vi "PantherLAB_Log - Duplicate DQMH Event.vi"(6 "Round Trip Broadcast Name":string, 7 "Destination Module":T1, 9 "New Event Name":string, 10 "Event Info (Existing)":T3={"Event VI Path"=path "", "Argument Path"=path "", "Wait Argument Path"=path "", "Event Arg Owner"=-1, "Event Name"="", "Type"=enum."Request"}, 11 "Source Module":T1) -> (0 "error out":errorcluster)   [LabVIEW 2016]
doc: "_____\nCreated using DQMH Framework: Event Scripter 7.1.0.1450."
uses:
  <vilib>/Delacor/Delacor QMH/Libraries/_Scripting Support/Module Info--cluster.ctl
  <vilib>/Delacor/Delacor QMH/Libraries/_Scripting Support/Module Type--enum.ctl
  <vilib>/Delacor/Delacor QMH/Libraries/_Scripting Support/Event Info (Existing)--cluster.ctl
  Program Files (x86)/National Instruments/LabVIEW 2016/project/Delacor/DQMH/_DQMH Remove Event/Event Type (All Permutations)--enum.ctl
  PantherLAB Scripting Hooks/PantherLAB_Scripting.lvlib
  <vilib>/Delacor/Delacor QMH/Libraries/_Scripting Support/dqmh_lib_DQMH Scripting Support.lvlib
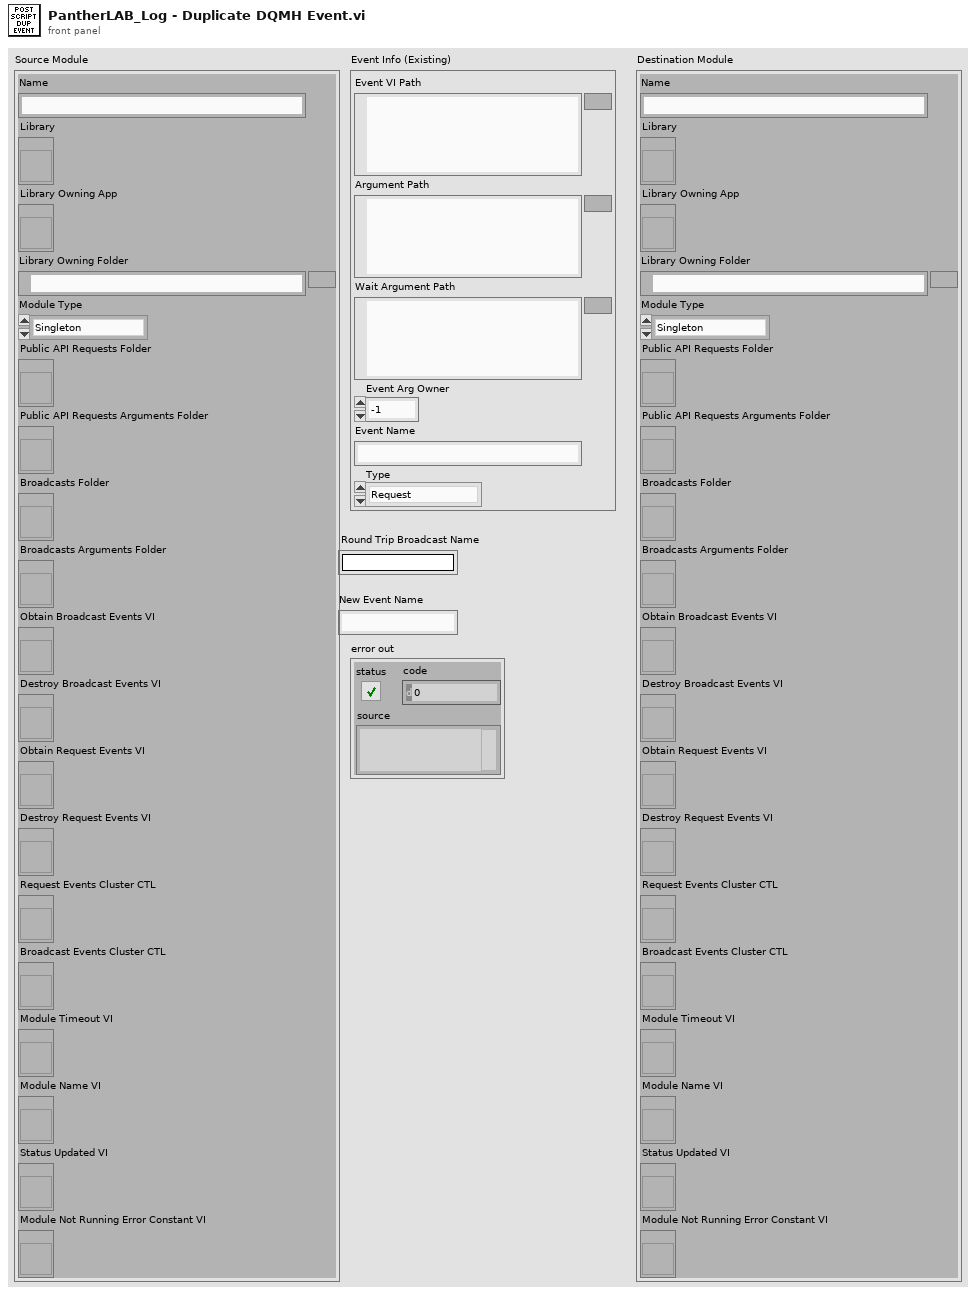
[diagram p1: front panel]
types:
  T1 = typedef "dqmh_lib_DQMH Scripting Support.lvlib/Module Info--cluster.ctl" = cluster{"Name":string, "Library":refnum<vi>, "Library Owning App":refnum<vi>, "Library Owning Folder":path, "Module Type":T2, "Public API Requests Folder":refnum<vi>, "Public API Requests Arguments Folder":refnum<vi>, "Broadcasts Folder":refnum<vi>, "Broadcasts Arguments Folder":refnum<vi>, "Obtain Broadcast Events VI":refnum<vi>, "Destroy Broadcast Events VI":refnum<vi>, "Obtain Request Events VI":refnum<vi>, "Destroy Request Events VI":refnum<vi>, "Request Events Cluster CTL":refnum<vi>, "Broadcast Events Cluster CTL":refnum<vi>, "Module Timeout VI":refnum<vi>, "Module Name VI":refnum<vi>, "Status Updated VI":refnum<vi>, "Module Not Running Error Constant VI":refnum<vi>}
  T2 = typedef "dqmh_lib_DQMH Scripting Support.lvlib/Module Type--enum.ctl" = enum16{"Singleton", "Cloneable"}
  T3 = typedef "dqmh_lib_DQMH Scripting Support.lvlib/Event Info (Existing)--cluster.ctl" = cluster{"Event VI Path":path, "Argument Path":path, "Wait Argument Path":path, "Event Arg Owner":i32, "Event Name":string, "Type":T4}
  T4 = typedef "dqmh_lib_DQMH Scripting Support.lvlib/Event Type (All Permutations)--enum.ctl" = enum16{"Request", "Broadcast", "Both", "Request (no Wait)", "Request and Wait", "Request (Private)", "Request (Local Instance)"}
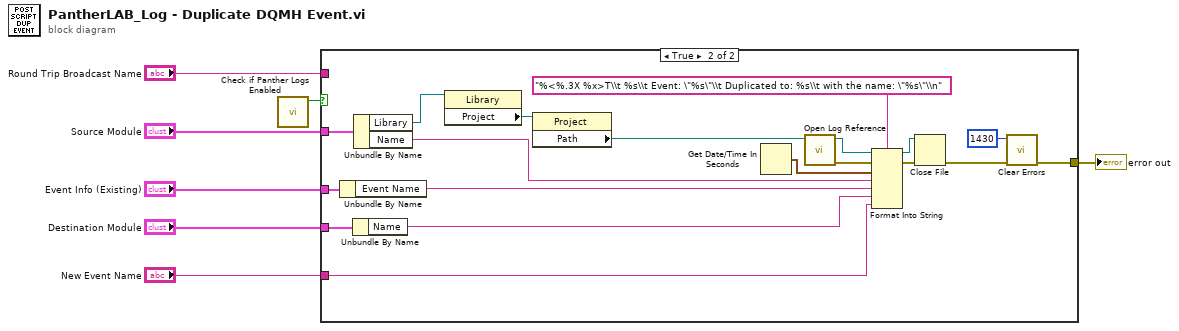
[diagram p0: block diagram]
diagram:
  n1 = call "Check if Panther Logs Enabled.vi"() -> ("PantherLogs Enabled?"=w6:bool)  [unwired: 11 in]
  n2 = case shown="True" w6 {
    tunnel: [_ w9] -> w7
    tunnel: "Source Module" -> [_ w23]
    tunnel: "Destination Module" -> [_ w13]
    tunnel: "Event Info (Existing)" -> [_ w15]
    tunnel: "New Event Name" -> [_ w11]
    tunnel: "Round Trip Broadcast Name" -> [_ _]
    frame False {
    }
    frame True {
      n3 = Unbundle By Name(w15) -> ("Event Name"=w14:string)
      n4 = Unbundle By Name(w13) -> ("Name"=w12:string)
      n5 = Unbundle By Name(w23) -> ("Library"=w22:refnum<vi>, "Name"=w18:string)
      n6 = property class="Library"(reference=w22) -> ("Project"=w21:refnum<vi>)  [unwired: 1 in, 2 out]
      n7 = property class="Project"(reference=w21) -> ("Path"=w16:path)  [unwired: 1 in, 2 out]
      n8 = Get Date/Time In Seconds() -> (seconds since 1Jan1904=w17:timestamp)
      n9 = call "Open Log Reference.vi"("Project Path"=w16) -> ("error out"=w26:errorcluster, "File Reference"=w20:refnum<file>)  [unwired: 9 in]
      n10 = Format Into String(format string="%<%.3X %x>T\\t %s\\t Event: \"%s\"\\t Duplicated to: %s\\t with the name: \"%s\"\\n", initial string=w20, error in=w26, w17, w18, w14, w12, w11) -> (resulting string=w19:refnum<file>, error out=w25:errorcluster)
      n11 = Close File(refnum=w19, error in=w25) -> (error out=w24:errorcluster)  [unwired: 1 out]
      n12 = call <vilib>:"Clear Errors.vi"("error in (no error)"=w24, "specific error code to clear (0: all)"=1430) -> ("error out"=w9:errorcluster)  [unwired: 4 in, 1 out]
    }
  }
  "error out" <- w7
